vi "testQueuesCommands.vi"(5 "QueueDisplay":refnum<queue>, 7 "QueueMessages":refnum<queue>, 8 "error in (no error)":errorcluster, 10 "newParam":T5 {"HoloParam"."Holo size X" format="%.0g"; "HoloParam"."pixel size" format="%#_6e"; "HoloParam"."wavelength" format="%#_6e"; "anaParam"."CCL parameters"."max voxel" min=0.0 max=0.0; "anaParam"."CCL parameters"."min voxel" min=1.0 max=100.0; "anaParam"."CCL parameters"."Threshold ( N x Standard deviation)" min=1.0 max=100.0; "anaParam"."Focus"."Sum size" min=1 max=100; "anaParam"."propagation"."Fourier BP filter (pix)"."Low Pass (0=none)" format="%#_6e"; "anaParam"."propagation"."step" format="%#_6e"; "anaParam"."propagation"."distance ini" format="%#_6e"}, 11 "DatasIN":T1={"PythonSession"=refnum, "Display"=FALSE, "BinThreshold"=0.0, "LIST HOLO BATCH"=[], "Display"=[], "meanHolo"=[], "FEATURES(µm)"=[], "LabelPicture"="", "Status"="", "planeToDisplayFeatures"=enum."XY", "State"=enum."WAIT"}) -> (0 "error out":errorcluster, 3 "DatasOUT":T1={"PythonSession"=refnum, "Display"=FALSE, "BinThreshold"=0.0, "LIST HOLO BATCH"=[], "Display"=[], "meanHolo"=[], "FEATURES(µm)"=[], "LabelPicture"="", "Status"="", "planeToDisplayFeatures"=enum."XY", "State"=enum."WAIT"})   [LabVIEW 2023]
uses:
  HoloPyLib/CCL_parameters.ctl
  analyse_parameters.ctl
  HoloPyLib/holoPyTracks.lvlib
  HologramInfo.ctl
  datas.ctl
  analyses_parameters.ctl
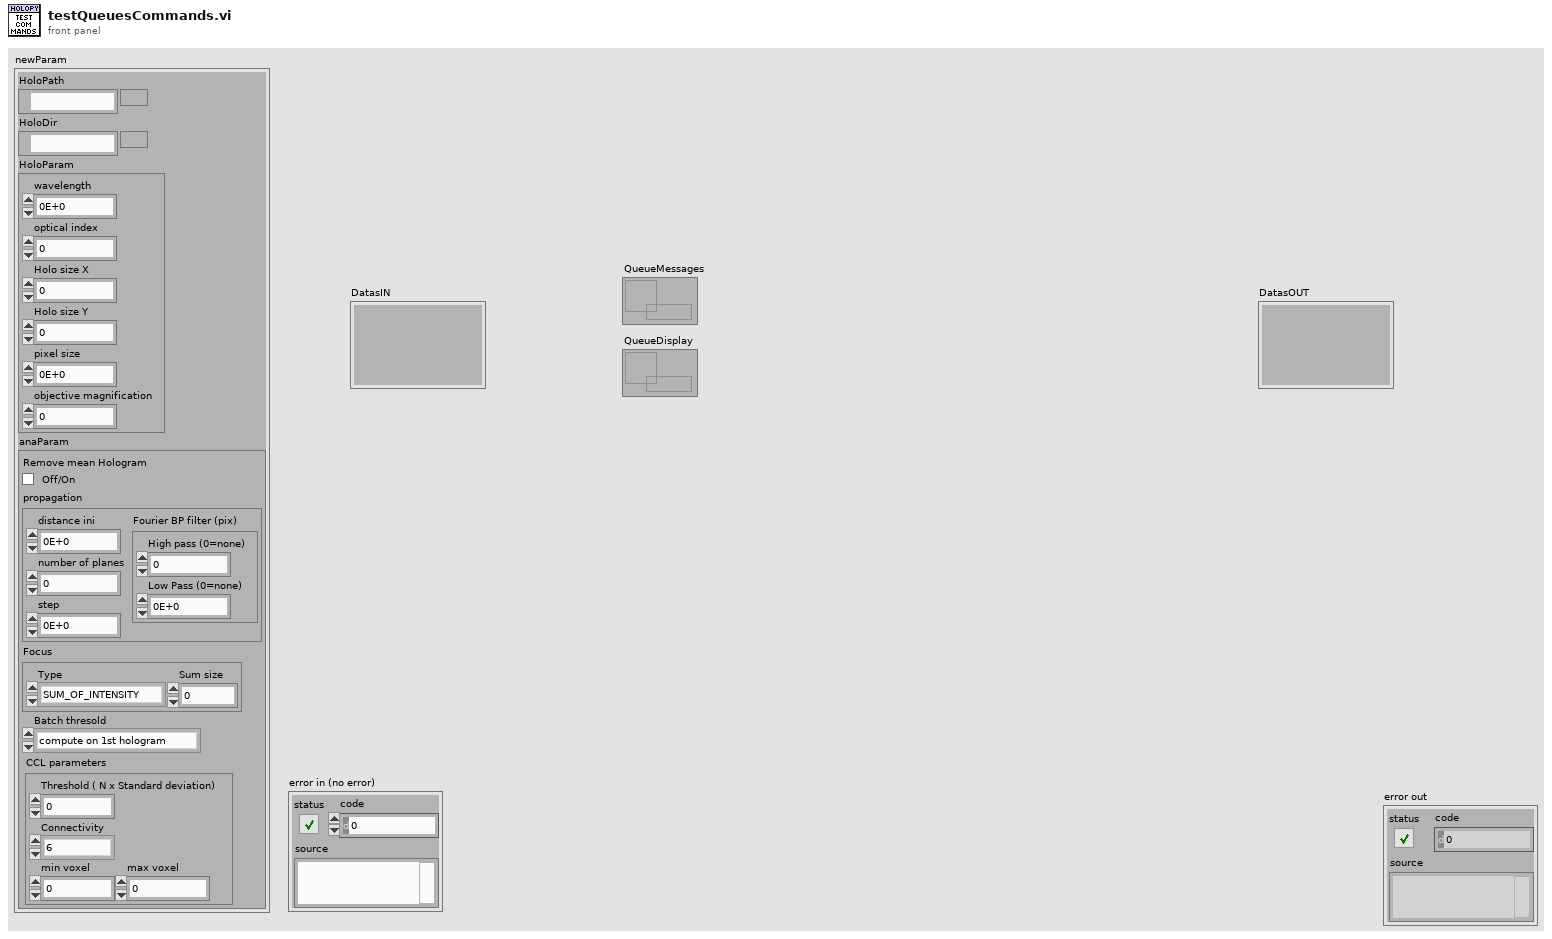
[diagram p1: front panel]
types:
  T1 = typedef "datas.ctl" = cluster{"PythonSession":refnum<k35>, "Display":bool, "BinThreshold":sgl, "LIST HOLO BATCH":path[], "Display":sgl[][], "meanHolo":sgl[][], "FEATURES(µm)":sgl[][], "LabelPicture":string, "Status":string, "planeToDisplayFeatures":enum16{"XY", "XZ", "YZ"}, "State":enum16{"SESSION CLOSED", "WAIT", "TEST WAIT", "TEST IN PROGESS", "BATCH IN PROGRESS"}}
  T2 = typedef "holoPyTracks.lvlib/HologramInfo.ctl" = cluster{"wavelength":sgl, "optical index":sgl, "Holo size X":i32, "Holo size Y":i32, "pixel size":sgl, "objective magnification":sgl}
  T3 = typedef "holoPyTracks.lvlib/analyses_parameters.ctl" = cluster{"propagation":cluster{"distance ini":dbl, "number of planes":i32, "step":dbl, "Fourier BP filter (pix)":cluster{"High pass (0=none)":dbl, "Low Pass (0=none)":dbl}}, "Focus":cluster{"Type":enum16{"SUM_OF_INTENSITY", "SUM_OF_LAPLACIAN", "SUM_OF_VARIANCE", "TENENGRAD"}, "Sum size":i32}, "Remove mean Hologram":bool, "CCL parameters":T4, "Batch thresold ":enum16{"compute on 1st hologram", "compute on each hologram"}}
  T4 = typedef "CCL_parameters.ctl" = cluster{"Threshold ( N x Standard deviation)":dbl, "Connectivity":enum16{"6", "18", "26"}, "min voxel":dbl, "max voxel":dbl}
  T5 = cluster{"HoloPath":path, "HoloDir":path, "HoloParam":T2, "anaParam":T3}
  T6 = typedef "holoPyTracks.lvlib/analyse_parameters.ctl" = cluster{"propagation":cluster{"distance ini":dbl, "number of planes":i32, "step":dbl, "Fourier BP filter (pix)":cluster{"High pass (0=none)":dbl, "Low Pass (0=none)":dbl}}, "Focus":cluster{"Type":enum16{"SUM_OF_INTENSITY", "SUM_OF_LAPLACIAN", "SUM_OF_VARIANCE", "TENENGRAD"}, "Sum size":i32}, "Remove mean Hologram":bool, "CCL parameters":T4}
  T7 = cluster{"distance ini":dbl, "number of planes":i32, "step":dbl, "Fourier BP filter (pix)":cluster{"High pass (0=none)":dbl, "Low Pass (0=none)":dbl}}
  T8 = cluster{"Type":enum16{"SUM_OF_INTENSITY", "SUM_OF_LAPLACIAN", "SUM_OF_VARIANCE", "TENENGRAD"}, "Sum size":i32}
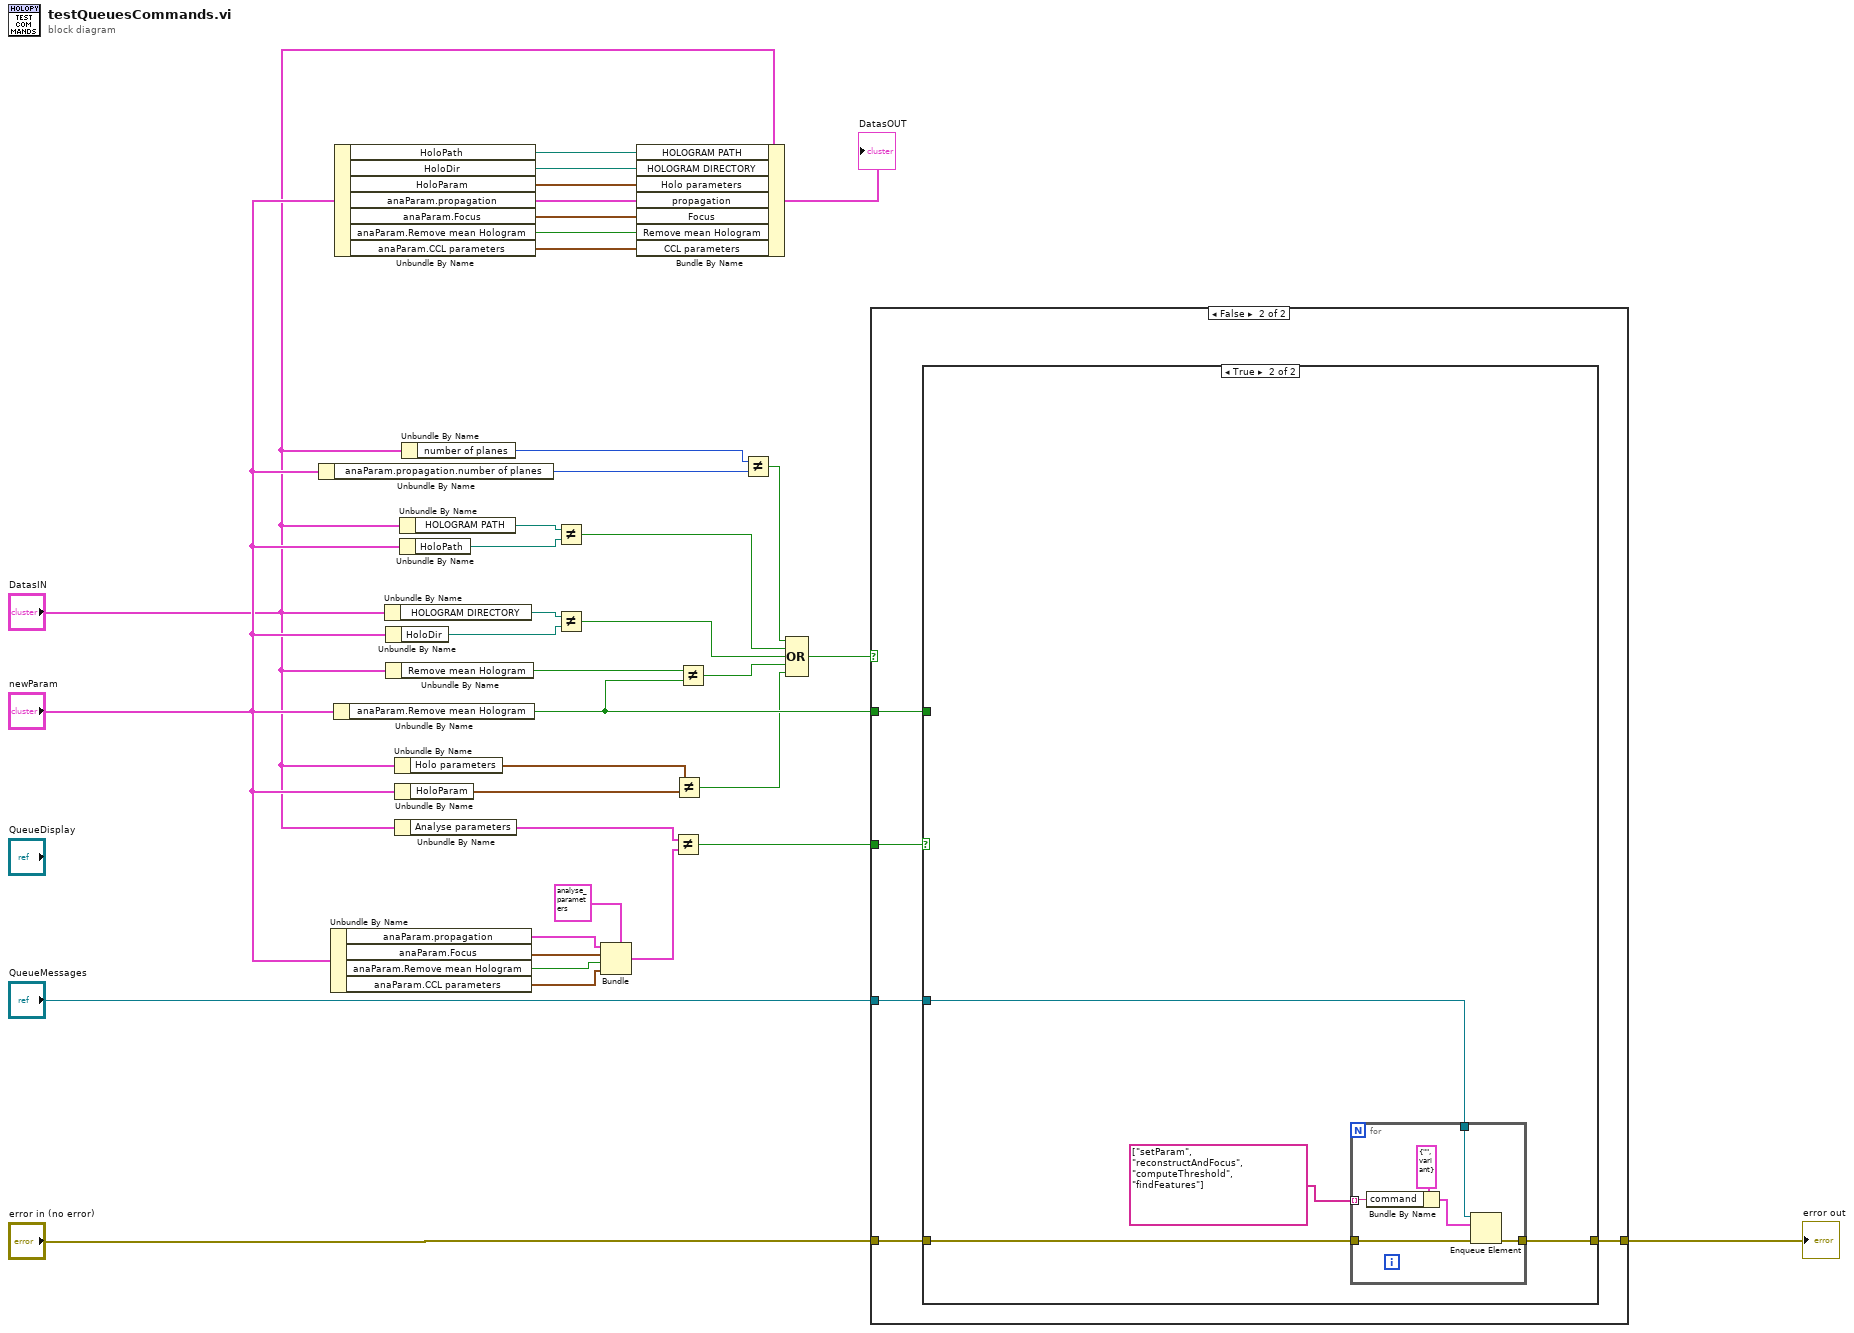
[diagram p0: block diagram]
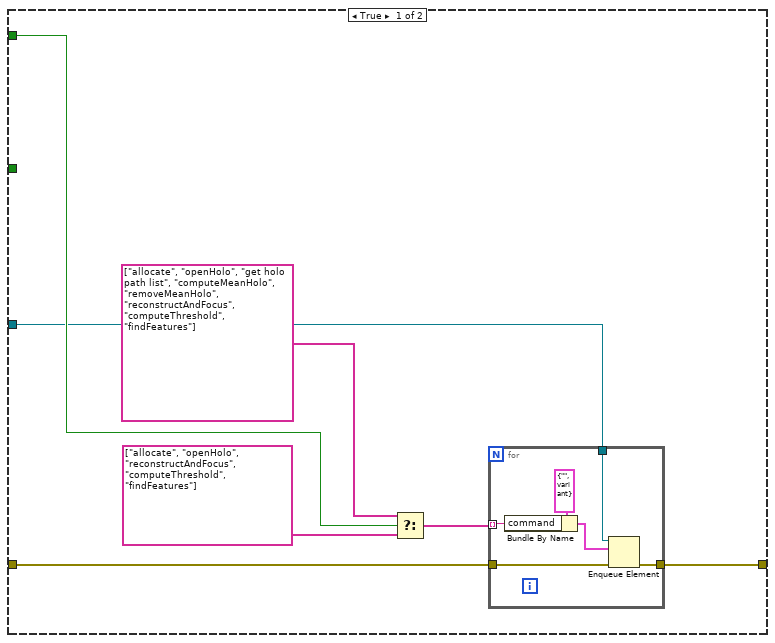
[diagram p2: hidden frame]
diagram:
  n1 = Unbundle By Name("newParam") -> ("anaParam.propagation.number of planes"=w32:i32)
  n2 = Unbundle By Name("newParam") -> ("anaParam.propagation"=w16:T7, "anaParam.Focus"=w15:T8, "anaParam.Remove mean Hologram"=w14:bool, "anaParam.CCL parameters"=w13:T4)
  n3 = Unbundle By Name("newParam") -> ("anaParam.Remove mean Hologram"=w29:bool)
  n4 = Unbundle By Name("newParam") -> ("HoloPath"=w7:path, "HoloDir"=w6:path, "HoloParam"=w5:T2, "anaParam.propagation"=w1:T7, "anaParam.Focus"=w2:T8, "anaParam.Remove mean Hologram"=w3:bool, "anaParam.CCL parameters"=w4:T4)
  n5 = Unbundle By Name("DatasIN") -> ("HOLOGRAM DIRECTORY"=w34:path)
  n6 = Unbundle By Name("newParam") -> ("HoloDir"=w35:path)
  n7 = Unbundle By Name("DatasIN") -> ("Remove mean Hologram"=w33:bool)
  n8 = Unbundle By Name("DatasIN") -> ("Holo parameters"=w21:T2)
  n9 = Unbundle By Name("newParam") -> ("HoloParam"=w20:T2)
  n10 = Unbundle By Name("DatasIN") -> ("Analyse parameters"=w18:T6)
  n11 = Unbundle By Name("DatasIN") -> ("HOLOGRAM PATH"=w37:path)
  n12 = Unbundle By Name("newParam") -> ("HoloPath"=w36:path)
  n13 = Unbundle By Name("DatasIN") -> ("number of planes"=w31:i32)
  n14 = Not Equal?(x=w37, y=w36) -> (x != y?=w24:bool)
  n15 = Not Equal?(x=w34, y=w35) -> (x != y?=w25:bool)
  n16 = Bundle(cluster=T6 {"propagation"={"distance ini"=0.0, "number of planes"=0, "step"=0.0, "Fourier BP filter (pix)"={"High pass (0=none)"=0.0, "Low Pass (0=none)"=0.0}}, "Focus"={"Type"=enum."SUM_OF_INTENSITY", "Sum size"=1}, "Remove mean Hologram"=FALSE, "CCL parameters"={"Threshold ( N x Standard deviation)"=10.0, "Connectivity"=enum."26", "min voxel"=1.0, "max voxel"=0.0}} ("Analyse parameters"), "propagation"=w16, "Focus"=w15, "Remove mean Hologram"=w14, "CCL parameters"=w13) -> (w12:T6)
  n17 = Bundle By Name(cluster="DatasIN", "HOLOGRAM PATH"=w7, "HOLOGRAM DIRECTORY"=w6, "Holo parameters"=w5, "propagation"=w1, "Focus"=w2, "Remove mean Hologram"=w3, "CCL parameters"=w4) -> (→"DatasOUT":T1)
  n18 = Not Equal?(x=w18, y=w12) -> (x != y?=w11:bool)
  n19 = Not Equal?(x=w21, y=w20) -> (x != y?=w19:bool)
  n20 = Not Equal?(x=w33, y=w29) -> (x != y?=w26:bool)
  n21 = Not Equal?(x=w31, y=w32) -> (x != y?=w23:bool)
  n22 = Compound Arithmetic op=OR(w23, w24, w25, w26, w19) -> (w22:bool)
  n23 = case shown="False" w22 {
    tunnel: "error in (no error)" -> [w42 w55]
    tunnel: w29 -> [w41 w54]
    tunnel: [w40 w53] -> w28
    tunnel: "QueueMessages" -> [w39 w52]
    tunnel: w11 -> [_ w51]
    frame True {
      n24 = Select(t=string[] ["allocate", "openHolo", "get holo path list", "computeMeanHolo", "removeMeanHolo", "reconstructAndFocus", "computeThreshold", "findFeatures"], s=w41, f=string[] ["allocate", "openHolo", "reconstructAndFocus", "computeThreshold", "findFeatures"]) -> (s? t:f=w44:string[])
      n25 = for {
        tunnel: w39 -> [w49]
        tunnel: w44 -> [w46] mode=indexing
        tunnel: w42 -> [w50]
        tunnel: [w48] -> w40
        n26 = Bundle By Name(cluster=cluster{"command":string, "data":variant} {"command"="", "data"=variant} ("element"), "command"=w46) -> (w45:cluster{"command":string, "data":variant})
        n27 = Enqueue Element(queue=w49, element=w45, error in (no error)=w50) -> (error out=w48:errorcluster)  [unwired: 1 in, 2 out]
      }
    }
    frame False {
      n28 = case shown="True" w51 {
        tunnel: w55 -> [w56 w60]
        tunnel: w54 -> [_ _]
        tunnel: [w56 w59] -> w53
        tunnel: w52 -> [_ w58]
        frame False {
        }
        frame True {
          n29 = for {
            tunnel: w58 -> [w65]
            tunnel: string[] ["setParam", "reconstructAndFocus", "computeThreshold", "findFeatures"] -> [w62] mode=indexing
            tunnel: w60 -> [w66]
            tunnel: [w64] -> w59
            n30 = Bundle By Name(cluster=cluster{"command":string, "data":variant} {"command"="", "data"=variant} ("element"), "command"=w62) -> (w61:cluster{"command":string, "data":variant})
            n31 = Enqueue Element(queue=w65, element=w61, error in (no error)=w66) -> (error out=w64:errorcluster)  [unwired: 1 in, 2 out]
          }
        }
      }
    }
  }
  "error out" <- w28
